vi "Init Horizontal.vi"(8 "error in (no error)":errorcluster, 11 "Tektronix MSO 6 Driver in":refnum<class "Tektronix MSO 6 Driver.lvclass">) -> (0 "error out":errorcluster, 3 "Tektronix MSO 6 Driver out":refnum<class "Tektronix MSO 6 Driver.lvclass">)   [LabVIEW 2021, in "Tektronix MSO 6 Driver.lvclass"]
uses:
  Tektronix MSO 6 Driver.lvclass
  Tektronix MSO 6 Driver.lvclass/Tektronix MSO 6 Driver.ctl
  <instrlib>/Tektronix MSO5X Series/Tektronix MSO5X Series.lvlib
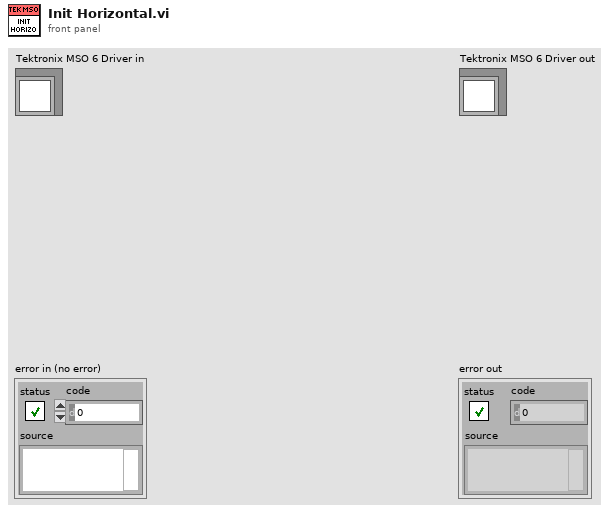
[diagram p1: front panel]
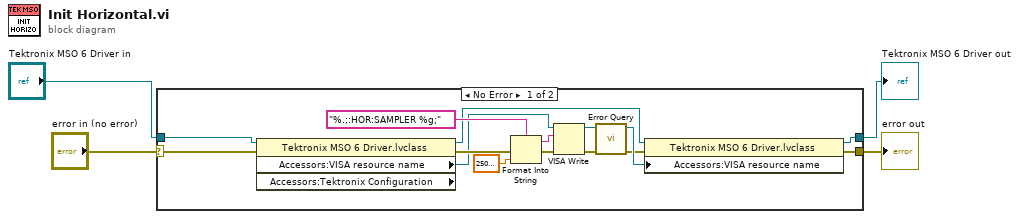
[diagram p0: block diagram]
diagram:
  n1 = case shown="No Error" "error in (no error)" {
    selector: "error in (no error)" -> [w10 w21]
    tunnel: [w7 w21] -> w3
    tunnel: [w6 w20] -> w1
    tunnel: "Tektronix MSO 6 Driver in" -> [w19 w20]
    frame No Error {
      n2 = property class="Tektronix MSO 6 Driver.lvclass" props=["Accessors:VISA resource name", "Accessors:Tektronix Configuration"](reference=w19, error in=w10) -> (reference out=w5:refnum<class "Tektronix MSO 6 Driver.lvclass">, error out=w17:errorcluster, "Accessors:VISA resource name"=w11:refnum<visa-resource-name>)  [unwired: 1 out]
      n3 = Format Into String(format string="%.;:HOR:SAMPLER %g;", error in=w17, 25000000000.0 ("Sample Rate (3.125E+9)")) -> (resulting string=w12:string, error out=w13:errorcluster)  [unwired: 1 in]
      n4 = VISA Write(VISA resource name=w11, write buffer=w12, error in (no error)=w13) -> (VISA resource name out=w14:refnum<visa-resource-name>, error out=w15:errorcluster)  [unwired: 1 out]
      n5 = call <instrlib>:"Error Query.vi"("error in (no error)"=w15, "VISA resource name"=w14) -> ("error out"=w8:errorcluster, "VISA resource name out"=w9:refnum<visa-resource-name>)  [unwired: 6 in, 2 out]
      n6 = property class="Tektronix MSO 6 Driver.lvclass"(reference=w5, error in=w8, "Accessors:VISA resource name"=w9) -> (reference out=w6:refnum<class "Tektronix MSO 6 Driver.lvclass">, error out=w7:errorcluster)
    }
    frame Error {
    }
  }
  "error out" <- w3
  "Tektronix MSO 6 Driver out" <- w1
